vi "SENS_FOM_RANG_NAME.vi"(0 "VISA IN":refnum<visa-resource-name>, 1 "Range number":i32, 5 "error in":errorcluster, 7 "Channel":i32) -> (14 "VISA Out":refnum<visa-resource-name>, 16 "Data":string, 19 "error out":errorcluster)   [LabVIEW 2018, in "PNA-X.lvlib"]
doc: "SENSe<cnum>:FOM:RANGe<n>:NAME? \n1741\n\n(Read-only) Returns the name of range<n>. \nThe FOM range items are typically named as follows: \nPrimary 1. \nSource 2. \nReceivers 3. \nSource2 (if present) 4. \nParameters \n<cnum> Any existing channel number; if unspecified, value is set to 1. \n<n> Range number. If unspecified, value is set to 1. \nExamples SENS:FOM:RANG:NAME? \nsense2:fom:range2:name? \nReturn Type String \nDefault Not Applicable"
uses:
  PNA-X.lvlib
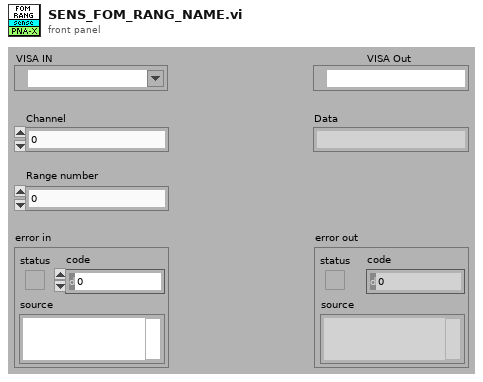
[diagram p1: front panel]
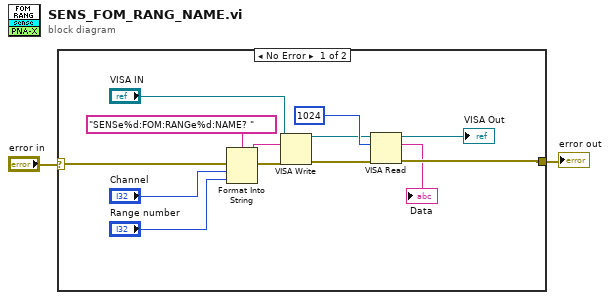
[diagram p0: block diagram]
diagram:
  n1 = case shown="No Error" "error in" {
    selector: "error in" -> [w15 w16]
    tunnel: [w6 w16] -> w1
    frame No Error {
      n2 = Format Into String(format string="SENSe%d:FOM:RANGe%d:NAME? " ("Cmdline"), error in=w15, "Channel", "Range number") -> (resulting string=w13:string, error out=w14:errorcluster)  [unwired: 1 in]
      n3 = VISA Write(VISA resource name="VISA IN", write buffer=w13, error in (no error)=w14) -> (VISA resource name out=w8:refnum<visa-resource-name>, error out=w10:errorcluster)  [unwired: 1 out]
      n4 = VISA Read(VISA resource name=w8, byte count=1024, error in (no error)=w10) -> (VISA resource name out=→"VISA Out":refnum<visa-resource-name>, read buffer=→"Data":string, error out=w6:errorcluster)  [unwired: 1 out]
    }
    frame Error {
    }
  }
  "error out" <- w1
